vi "FRCts20_EspEngine_Reports_SwUsage.vi"(8 "error in (no error)":errorcluster, 10 "Software Usage Pie":T1, 11 "httpRequestID":u32) -> (0 "error out":errorcluster, 3 "httpRequestID out":u32)   [LabVIEW 2014, in "FRCts20_EspEngine.lvlib"]
uses:
  FRCts20_EspEngine.lvlib
  TypeDefs/FRCts20_EspEngine_SwUsage_Pie.ctl
  <vilib>/wsapi/subVIs/Set Integer ESP Variable.vi
  FRCts20_EspEngine_FormatArrayOfKeysStrings.vi
  FRCts20_EspEngine_FormatArrayOfKeysDbls.vi
  FRCts20_EspEngine_FormatArrayOfKeysInts.vi
  <vilib>/wsapi/NI_WebServices.lvlib
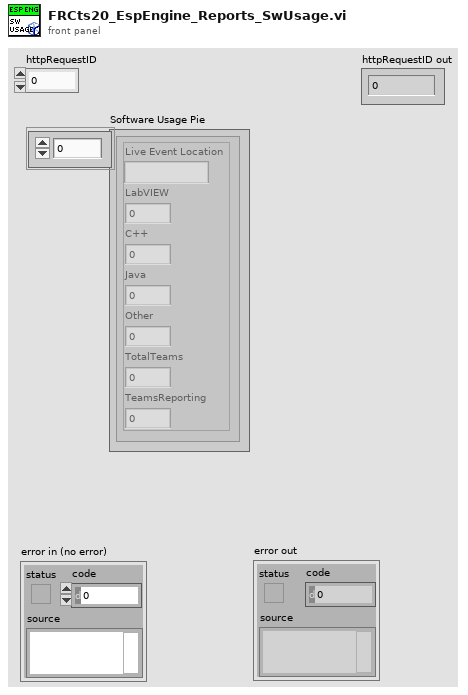
[diagram p1: front panel]
types:
  T1 = typedef "FRCts20_EspEngine.lvlib/FRCts20_EspEngine_SwUsage_Pie.ctl" = cluster{"Live Event Location":string, "LabVIEW":dbl, "C++":dbl, "Java":dbl, "Other":dbl, "TotalTeams":i32, "TeamsReporting":i32}[]
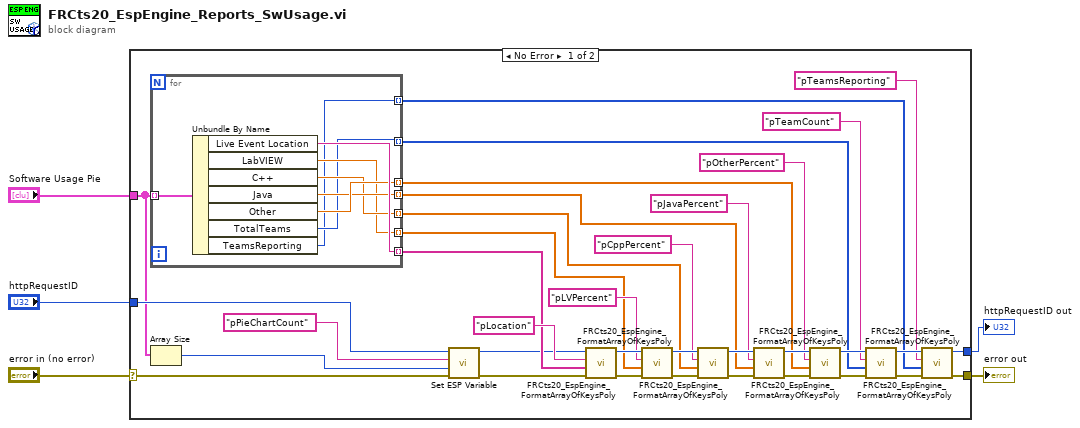
[diagram p0: block diagram]
diagram:
  n1 = case shown="No Error" "error in (no error)" {
    selector: "error in (no error)" -> [w19 w49]
    tunnel: [w7 w49] -> w5
    tunnel: "Software Usage Pie" -> [w17 _]
    tunnel: "httpRequestID" -> [w21 _]
    tunnel: [w6 _] -> w1
    frame No Error {
      n2 = for {
        tunnel: w17 -> [w48] mode=indexing
        tunnel: [w47] -> w30 mode=indexing
        tunnel: [w46] -> w26 mode=indexing
        tunnel: [w45] -> w25 mode=indexing
        tunnel: [w44] -> w24 mode=indexing
        tunnel: [w43] -> w23 mode=indexing
        tunnel: [w42] -> w9 mode=indexing
        tunnel: [w41] -> w8 mode=indexing
        n3 = Unbundle By Name(w48) -> ("Live Event Location"=w47:string, "LabVIEW"=w43:dbl, "C++"=w44:dbl, "Java"=w45:dbl, "Other"=w46:dbl, "TotalTeams"=w42:i32, "TeamsReporting"=w41:i32)
      }
      n4 = Array Size(array=w17) -> (size(s)=w16:i32)
      n5 = call-poly <vilib>:"Set ESP Variable.vi"("error in (no error)"=w19, "value"=w16, "key"="pPieChartCount", "httpRequestID"=w21) -> ("error out"=w18:errorcluster, "httpRequestID out"=w20:u32)  [unwired: 6 in]
      n6 = call-poly "FRCts20_EspEngine_FormatArrayOfKeysPoly.vi"("error IO"=w18, "Values"=w30, "KeyBaseName"="pLocation", "httpRequestID"=w20) -> ("error IO"=w40:errorcluster, "httpRequestID out"=w39:u32)  [unwired: 6 in]
      n7 = call-poly "FRCts20_EspEngine_FormatArrayOfKeysPoly.vi"("error IO"=w40, "Values"=w23, "KeyBaseName"="pLVPercent", "httpRequestID"=w39) -> ("error IO"=w38:errorcluster, "httpRequestID out"=w37:u32)  [unwired: 6 in]
      n8 = call-poly "FRCts20_EspEngine_FormatArrayOfKeysPoly.vi"("error IO"=w38, "Values"=w24, "KeyBaseName"="pCppPercent", "httpRequestID"=w37) -> ("error IO"=w36:errorcluster, "httpRequestID out"=w35:u32)  [unwired: 6 in]
      n9 = call-poly "FRCts20_EspEngine_FormatArrayOfKeysPoly.vi"("error IO"=w36, "Values"=w25, "KeyBaseName"="pJavaPercent", "httpRequestID"=w35) -> ("error IO"=w29:errorcluster, "httpRequestID out"=w28:u32)  [unwired: 6 in]
      n10 = call-poly "FRCts20_EspEngine_FormatArrayOfKeysPoly.vi"("error IO"=w29, "Values"=w26, "KeyBaseName"="pOtherPercent", "httpRequestID"=w28) -> ("error IO"=w11:errorcluster, "httpRequestID out"=w15:u32)  [unwired: 6 in]
      n11 = call-poly "FRCts20_EspEngine_FormatArrayOfKeysPoly.vi"("error IO"=w11, "Values"=w9, "KeyBaseName"="pTeamCount", "httpRequestID"=w15) -> ("error IO"=w10:errorcluster, "httpRequestID out"=w14:u32)  [unwired: 6 in]
      n12 = call-poly "FRCts20_EspEngine_FormatArrayOfKeysPoly.vi"("error IO"=w10, "Values"=w8, "KeyBaseName"="pTeamsReporting", "httpRequestID"=w14) -> ("error IO"=w7:errorcluster, "httpRequestID out"=w6:u32)  [unwired: 6 in]
    }
    frame Error {
    }
  }
  "error out" <- w5
  "httpRequestID out" <- w1
